vi "lv_mysql_conn_query.vi"(8 "error in (no error)":errorcluster, 9 "timeout ms (5000)":i32=5000, 10 "Query":string, 11 "connection ID":refnum<k5>) -> (0 "error out":errorcluster, 1 "Return Data":variant[][](array[variant]), 2 "Packet Metadata":T1 {"Server Status" format="%.0x"}, 3 "connection ID out":refnum<k5>)   [LabVIEW 2020]
uses:
  Control/ok_packet_metadata.ctl
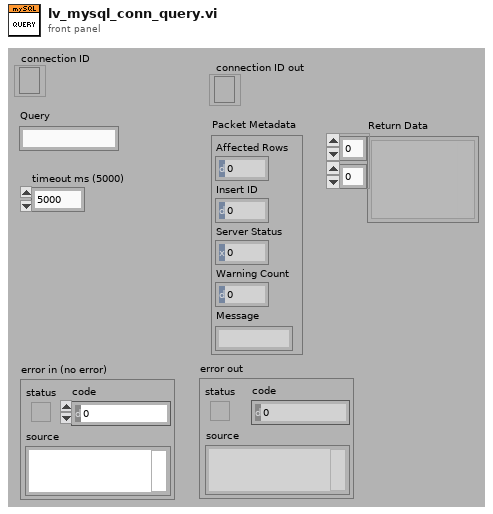
[diagram p1: front panel]
types:
  T1 = typedef "ok_packet_metadata.ctl" = cluster{"Affected Rows":u64, "Insert ID":u64, "Server Status":u16, "Warning Count":u16, "Message":string}
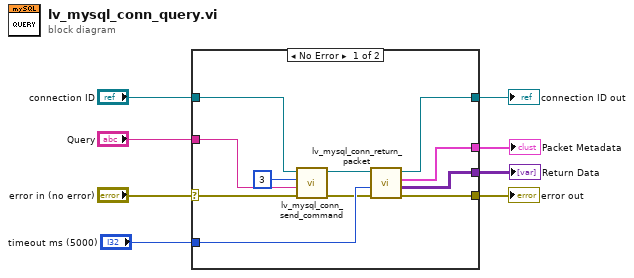
[diagram p0: block diagram]
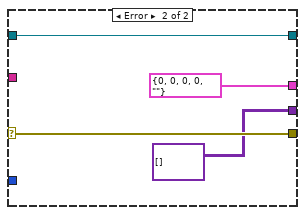
[diagram p2: hidden frame]
diagram:
  n1 = case shown="No Error" "error in (no error)" {
    selector: "error in (no error)" -> [w17 w23]
    tunnel: [w15 w23] -> w7
    tunnel: [w13 w22] -> w6
    tunnel: "connection ID" -> [w16 w22]
    tunnel: "Query" -> [w19 _]
    tunnel: "timeout ms (5000)" -> [w12 _]
    tunnel: [w14 variant[][] [] ("Return Data")] -> w2
    tunnel: [w11 T1 {"Affected Rows"=0, "Insert ID"=0, "Server Status"=0, "Warning Count"=0, "Message"=""} ("Packet Metadata")] -> w1
    frame No Error {
      n2 = call "lv_mysql_conn_send_command.vi"("error in (no error)"=w17, "Message"=w19, "Command"=u8 3, "connection ID"=w16) -> ("error out"=w9:errorcluster, "connection ID out"=w10:refnum<k5>)  [unwired: 6 in]
      n3 = call "lv_mysql_conn_return_packet.vi"("error in (no error)"=w9, "timeout ms (5000)"=w12, "connection ID"=w10) -> ("error out"=w15:errorcluster, "Return Data"=w14:variant[][], "Packet Metadata"=w11:T1, "connection ID out"=w13:refnum<k5>)  [unwired: 5 in]
    }
    frame Error {
    }
  }
  "error out" <- w7
  "connection ID out" <- w6
  "Return Data" <- w2
  "Packet Metadata" <- w1
